vi "Initialization VI.vi"(8 "error in (no error)":errorcluster, 10 "Custom XML":string, 11 "Device Item Ref in":T1 format="%.0x") -> (0 "error out":errorcluster, 3 "Device Item Ref out":T1 format="%.0x")   [LabVIEW 2019, in "Ghost Bus Addon System Explorer.lvlib"]
uses:
  Ghost Bus Addon System Explorer.lvlib
  <vilib>/NI VeriStand/Custom Device API/Custom Device API.lvlib
  Addon Shared/SubVIs/GUID Lookup.vi
  Addon Shared/Ghost Bus Addon Shared.lvlib
  <vilib>/NI VeriStand/Custom Device API/Custom Device Channel Type.ctl
  <vilib>/NI VeriStand/Custom Device API/Custom Device Channel.ctl
  <vilib>/NI VeriStand/Custom Device API/Custom Device Item Ref.ctl
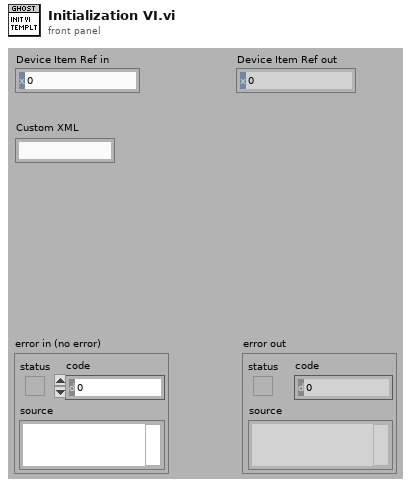
[diagram p1: front panel]
types:
  T1 = typedef "Custom Device API.lvlib/Custom Device Item Ref.ctl" = u64
  T2 = typedef "Custom Device API.lvlib/Custom Device Channel.ctl" = cluster{"Type":T3, "Units":string, "Default Value":dbl, "Faultable":bool, "Scalable":bool}
  T3 = typedef "Custom Device API.lvlib/Custom Device Channel Type.ctl" = enum16{"Input", "Output"}
  T4 = typedef "Ghost Bus Addon Shared.lvlib/XNET Settings.ctl" = cluster{"Database":refnum<k21>, "Cluster":refnum<k21>, "Primary":T5, "Ghost":T5}
  T5 = typedef "Ghost Bus Addon Shared.lvlib/XNET Port Settings.ctl" = cluster{"Port":string, "Baud Rate":u64, "Termination":u32, "CAN I/O Mode":u32, "FD Baud Rate":u64, "Priority":i32, "FD ISO Mode":u32}
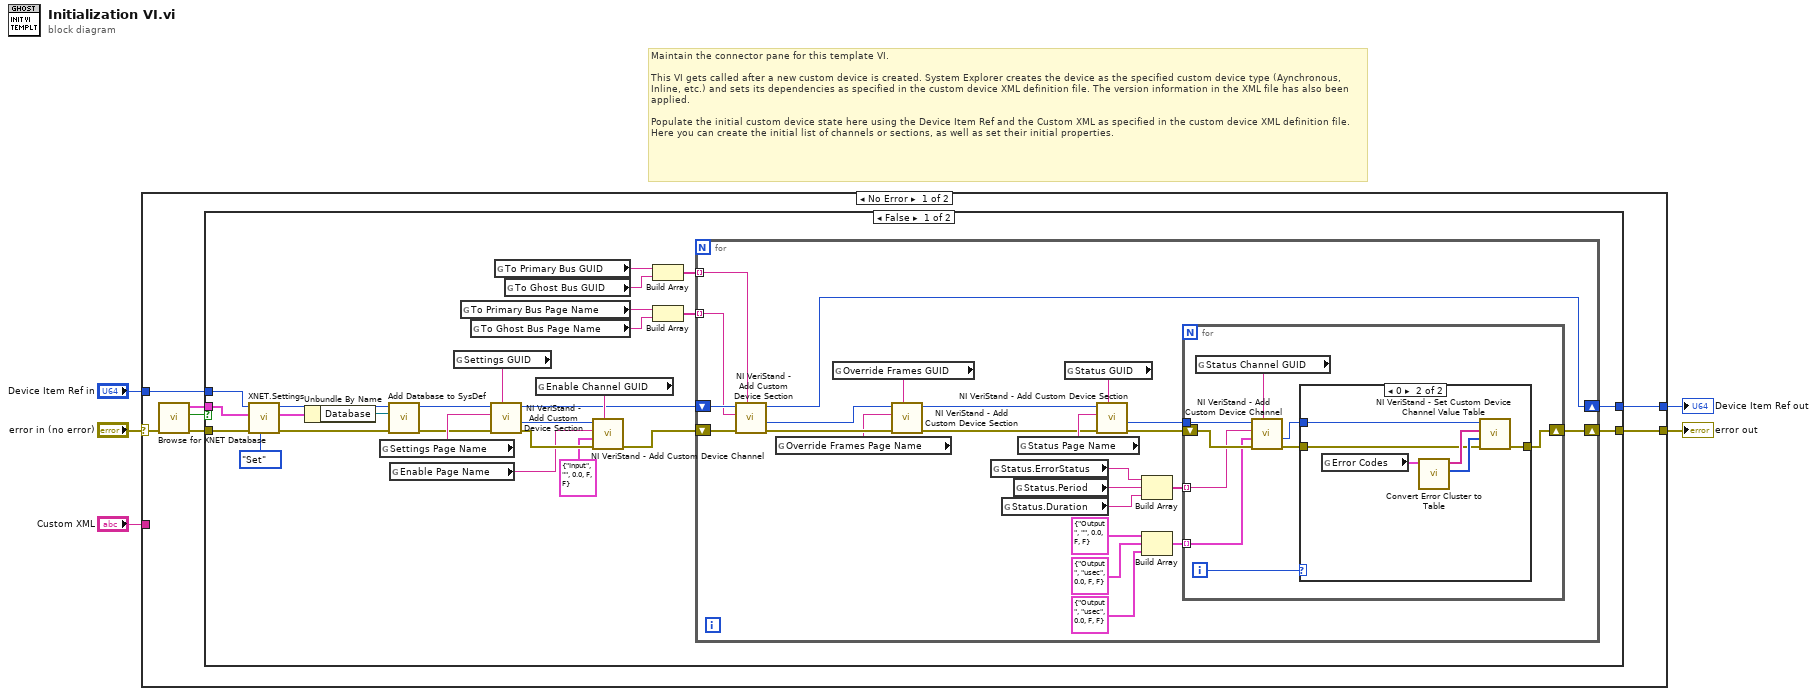
[diagram p0: block diagram]
diagram:
  # "Maintain the connector pane for this template VI.\n\nThis VI gets called after a new custom device is created. System Explorer creates the device as the specified custom device type (Aynchronous, Inline, etc.) and sets its dependencies as specified in the custom device XML definition file. The version information in the XML file has also been applied.\n\nPopulate the initial custom device state here using the Device Item Ref and the Custom XML as specified in the custom device XML definition file. Here you can create the initial list of channels or sections, as well as set their initial properties."
  n1 = case shown="No Error" "error in (no error)" {
    selector: "error in (no error)" -> [w10 w82]
    tunnel: [w12 w82] -> w5
    tunnel: [w11 w81] -> w3
    tunnel: "Device Item Ref in" -> [w8 w81]
    tunnel: "Custom XML" -> [_ _]
    frame No Error {
      n2 = call "Browse for XNET Database.vi"("error in (no error)"=w10) -> ("error out"=w9:errorcluster, "Cancel Out"=w7:bool, "XNET Settings"=w6:T4)  [unwired: 8 in]
      n3 = case shown="False" w7 {
        tunnel: [w30 w80] -> w12
        tunnel: [w31 w79] -> w11
        tunnel: w9 -> [w39 w80]
        tunnel: w8 -> [w37 w79]
        tunnel: w6 -> [w35 _]
        frame False {
          n4 = call "XNET.Settings.vi"("Action"=enum8{"Get", "Set"}."Set", "error in (no error)"=w39, "XNET Settings"=w35, "Parent Ref in"=w37) -> ("error out"=w38:errorcluster, "XNET Settings"=w34:T4, "Item Ref out"=w36:T1)  [unwired: 5 in]
          n5 = Unbundle By Name(w34) -> ("Database"=w33:refnum<k21>)
          n6 = global read "GUID Lookup.vi" "Settings Page Name"() -> (w23:string)
          n7 = call "Add Database to SysDef.vi"("error in"=w38, "DB Alias"=w33, "Item Ref in"=w36) -> ("error out"=w22:errorcluster, "Item Ref out"=w21:T1)  [unwired: 7 in]
          n8 = global read "GUID Lookup.vi" "Enable Page Name"() -> (w24:string)
          n9 = global read "GUID Lookup.vi" "Settings GUID"() -> (w26:string)
          n10 = global read "GUID Lookup.vi" "To Primary Bus Page Name"() -> (w18:string)
          n11 = global read "GUID Lookup.vi" "To Ghost Bus Page Name"() -> (w17:string)
          n12 = call <vilib>:"NI VeriStand - Add Custom Device Section.vi"("GUID (Default Section)"=w26, "error in (no error)"=w22, "Section Name"=w23, "Parent Ref in"=w21) -> ("error out"=w29:errorcluster, "Section Ptr"=w25:T1, "Parent Ref out"=w19:T1)  [unwired: 4 in, 1 out]
          n13 = global read "GUID Lookup.vi" "To Primary Bus GUID"() -> (w16:string)
          n14 = global read "GUID Lookup.vi" "To Ghost Bus GUID"() -> (w15:string)
          n15 = global read "GUID Lookup.vi" "Enable Channel GUID"() -> (w28:string)
          n16 = call <vilib>:"NI VeriStand - Add Custom Device Channel.vi"("GUID (Default Channel)"=w28, "error in (no error)"=w29, "Channel"=T2 {"Type"=enum."Input", "Units"="", "Default Value"=0.0, "Faultable"=FALSE, "Scalable"=FALSE}, "Channel Name"=w24, "Parent Ref in"=w25) -> ("error out"=w20:errorcluster)  [unwired: 3 in, 3 out]
          n17 = Build Array(w16, w15) -> (w13:string[])
          n18 = Build Array(w18, w17) -> (w14:string[])
          n19 = for {
            shift-right: [w60] -> w30
            shift-left: w20 -> [w49]
            shift-right: [w46] -> w31
            shift-left: w19 -> [w48]
            tunnel: w14 -> [w45] mode=indexing
            tunnel: w13 -> [w44] mode=indexing
            n20 = call <vilib>:"NI VeriStand - Add Custom Device Section.vi"("GUID (Default Section)"=w44, "error in (no error)"=w49, "Section Name"=w45, "Parent Ref in"=w48) -> ("error out"=w47:errorcluster, "Section Ptr"=w40:T1, "Parent Ref out"=w46:T1)  [unwired: 4 in, 1 out]
            n21 = global read "GUID Lookup.vi" "Override Frames Page Name"() -> (w43:string)
            n22 = global read "GUID Lookup.vi" "Override Frames GUID"() -> (w42:string)
            n23 = call <vilib>:"NI VeriStand - Add Custom Device Section.vi"("GUID (Default Section)"=w42, "Section Name"=w43, "Parent Ref in"=w40) -> ("Parent Ref out"=w41:T1)  [unwired: 5 in, 3 out]
            n24 = global read "GUID Lookup.vi" "Status.ErrorStatus"() -> (w59:string)
            n25 = global read "GUID Lookup.vi" "Status.Duration"() -> (w57:string)
            n26 = global read "GUID Lookup.vi" "Status.Period"() -> (w58:string)
            n27 = global read "GUID Lookup.vi" "Status Page Name"() -> (w54:string)
            n28 = global read "GUID Lookup.vi" "Status GUID"() -> (w55:string)
            n29 = call <vilib>:"NI VeriStand - Add Custom Device Section.vi"("GUID (Default Section)"=w55, "error in (no error)"=w47, "Section Name"=w54, "Parent Ref in"=w41) -> ("error out"=w61:errorcluster, "Section Ptr"=w62:T1)  [unwired: 4 in, 2 out]
            n30 = Build Array(w59, w58, w57) -> (w56:string[])
            n31 = Build Array(T2 {"Type"=enum."Output", "Units"="", "Default Value"=0.0, "Faultable"=FALSE, "Scalable"=FALSE} ("Channel"), T2 {"Type"=enum."Output", "Units"="usec", "Default Value"=0.0, "Faultable"=FALSE, "Scalable"=FALSE} ("Channel"), T2 {"Type"=enum."Output", "Units"="usec", "Default Value"=0.0, "Faultable"=FALSE, "Scalable"=FALSE} ("Channel")) -> (w50:T2[])
            n32 = for {
              tunnel: w62 -> [w71]
              shift-right: [w64] -> w60
              shift-left: w61 -> [w70]
              tunnel: w56 -> [w68] mode=indexing
              tunnel: w50 -> [w67] mode=indexing
              i -> [w66]
              n33 = global read "GUID Lookup.vi" "Status Channel GUID"() -> (w69:string)
              n34 = call <vilib>:"NI VeriStand - Add Custom Device Channel.vi"("GUID (Default Channel)"=w69, "error in (no error)"=w70, "Channel"=w67, "Channel Name"=w68, "Parent Ref in"=w71) -> ("error out"=w65:errorcluster, "Channel Ref"=w63:T1)  [unwired: 3 in, 2 out]
              n35 = case shown="0" w66 {
                tunnel: w63 -> [_ w77]
                tunnel: w65 -> [w72 w74]
                tunnel: [w72 w73] -> w64
                frame Default {
                }
                frame 0 {
                  n36 = global read "GUID Lookup.vi" "Error Codes"() -> (w78:cluster{"number":i32, "trimmed string":string}[])
                  n37 = call "Convert Error Cluster to Table.vi"("Error Codes"=w78) -> ("Code"=w75:i32[], "String"=w76:string[])  [unwired: 9 in]
                  n38 = call <vilib>:"NI VeriStand - Set Custom Device Channel Value Table.vi"("error in (no error)"=w74, "Values"=w75, "Names"=w76, "Channel Ref in"=w77) -> ("error out"=w73:errorcluster)  [unwired: 6 in, 1 out]
                }
              }
            }
          }
        }
        frame True {
        }
      }
    }
    frame Error {
    }
  }
  "error out" <- w5
  "Device Item Ref out" <- w3
